vi "PXI Multipliers to AO Gains (scalar).vi"(0 "Multiplier In":dbl, 11 "error in (no error)":errorcluster) -> (4 "Multiplier Out":dbl, 6 "Gain":dbl, 15 "error out":errorcluster)   [LabVIEW 2020]
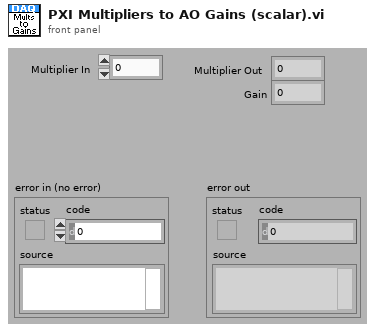
[diagram p1: front panel]
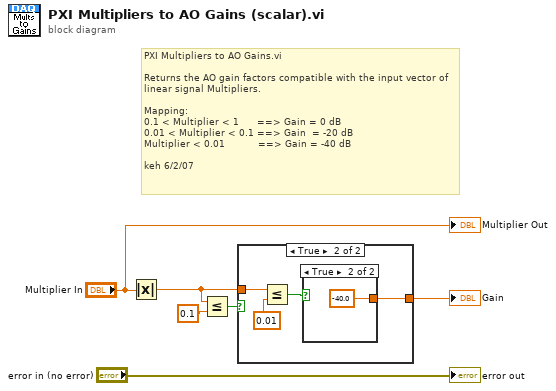
[diagram p0: block diagram]
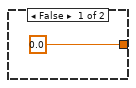
[diagram p2: hidden frame]
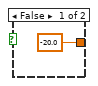
[diagram p3: hidden frame]
diagram:
  # "PXI Multipliers to AO Gains.vi\n\nReturns the AO gain factors compatible with the input vector of linear signal Multipliers.\n\nMapping:\n0.1 < Multiplier < 1      ==> Gain = 0 dB\n0.01 < Multiplier < 0.1 ==> Gain  = -20 dB\nMultiplier < 0.01           ==> Gain = -40 dB\n\nkeh 6/2/07"
  n1 = Absolute Value(x="Multiplier In") -> (abs(x)=w6:dbl)
  n2 = Less Or Equal?(x=w6, y=0.1) -> (x <= y?=w3:bool)
  n3 = case shown="True" w3 {
    tunnel: [0.0 w8] -> w2
    tunnel: w6 -> [_ w11]
    frame False {
    }
    frame True {
      n4 = Less Or Equal?(x=w11, y=0.01) -> (x <= y?=w9:bool)
      n5 = case shown="True" w9 {
        tunnel: [-20.0 ("y") -40.0 ("y")] -> w8
        frame False {
        }
        frame True {
        }
      }
    }
  }
  "Gain" <- w2
  "error out" <- "error in (no error)"
  "Multiplier Out" <- "Multiplier In"
